vi "GetCurrentPositionDegree.vi"(0 "StepMotor in":refnum<class "StepMotor.lvclass">, 5 "Редукция":dbl, 9 "Разрешение энкодера":dbl, 11 "error in (no error)":errorcluster) -> (4 "StepMotor out":refnum<class "StepMotor.lvclass">, 6 "Значение":dbl, 8 "RawPosition":dbl, 10 "360 и 0":bool, 15 "error out":errorcluster)   [LabVIEW 2010, in "StepMotor.lvclass"]
uses:
  StepMotor.lvclass
panel:
  out "RawPreviousPosition":dbl
  out "МножПриведШкалы360":dbl
  out "КолИмпулОборот":dbl
  out "Текущая позиция":dbl
  out "Инкремент импульсов":dbl
  out "Предыдущая позиция":dbl
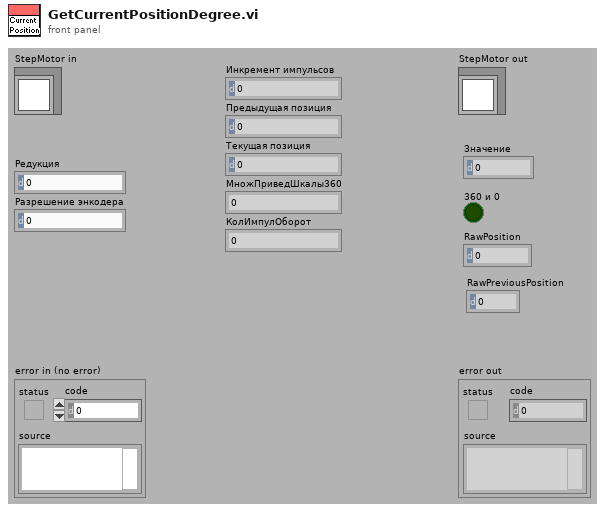
[diagram p1: front panel]
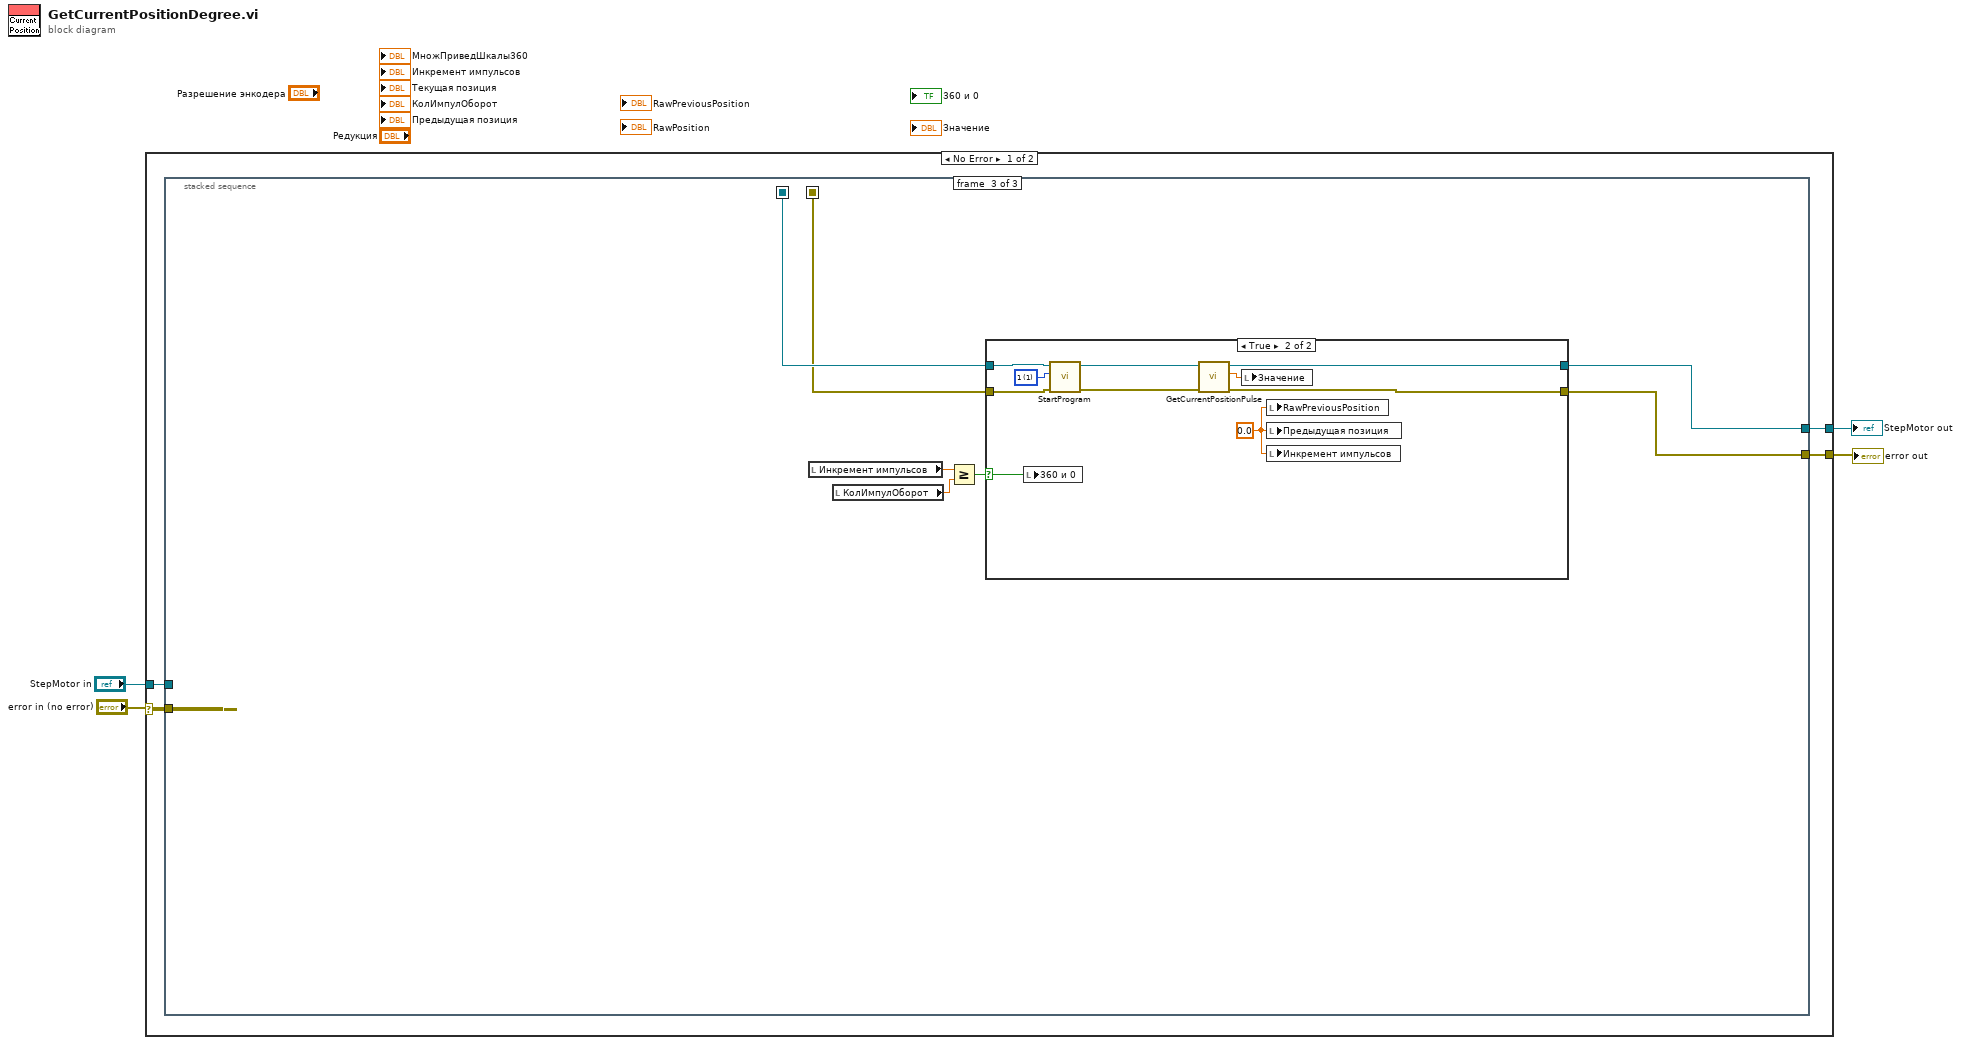
[diagram p0: block diagram]
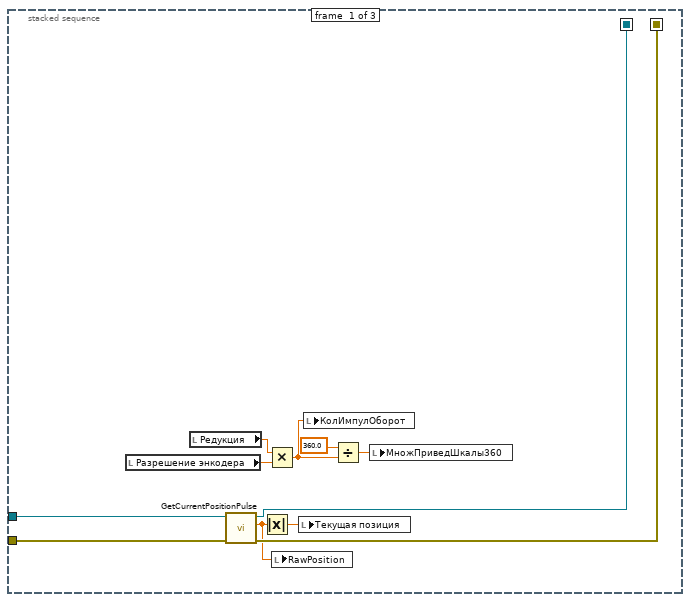
[diagram p2: hidden frame]
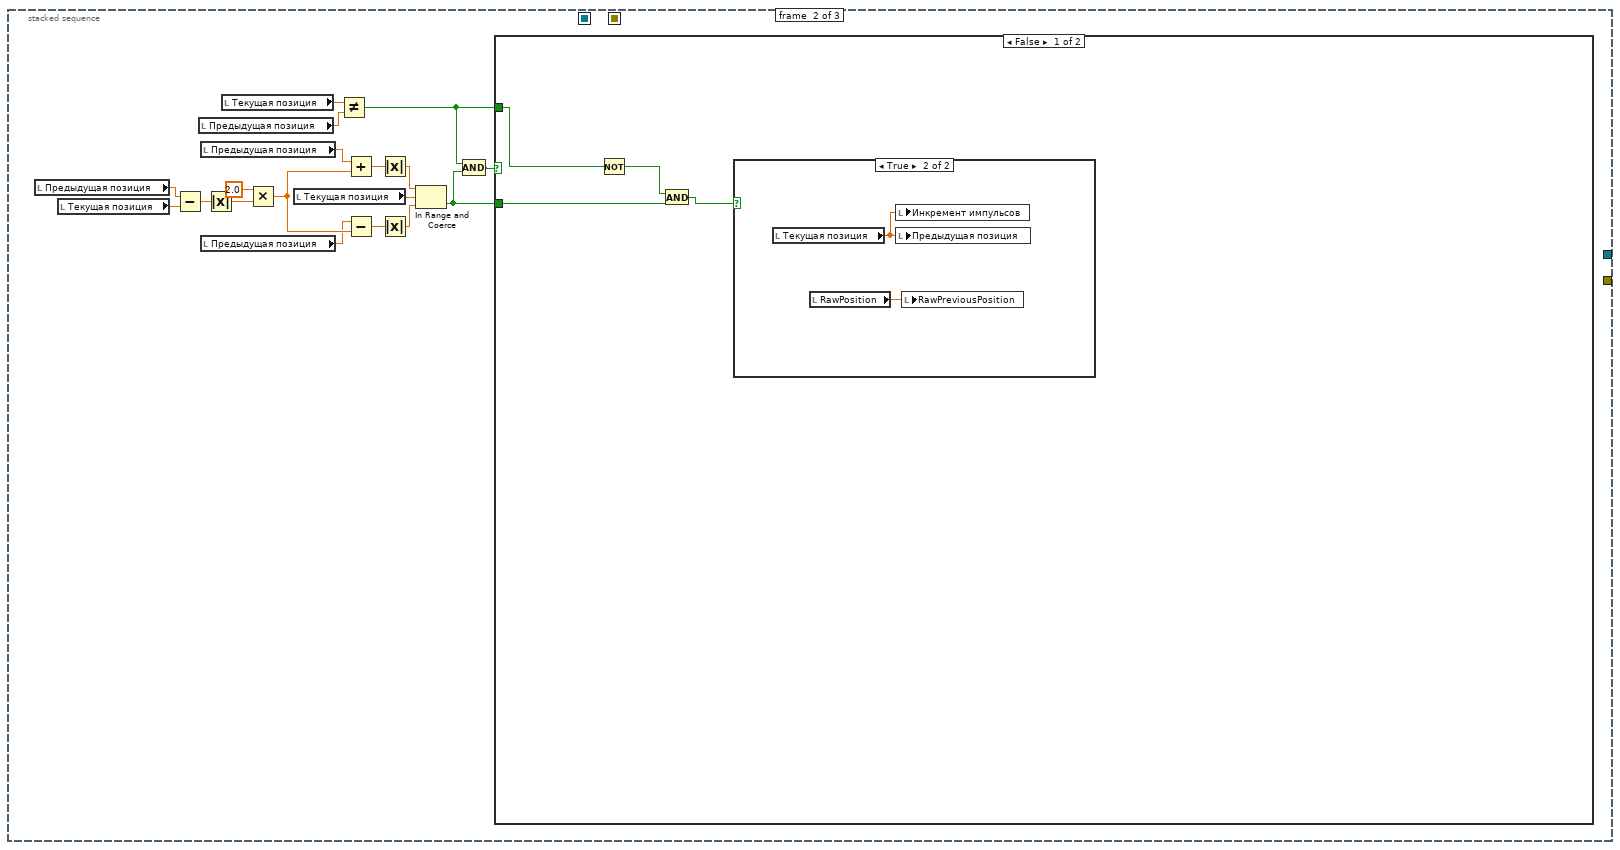
[diagram p3: hidden frame]
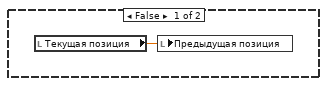
[diagram p4: hidden frame]
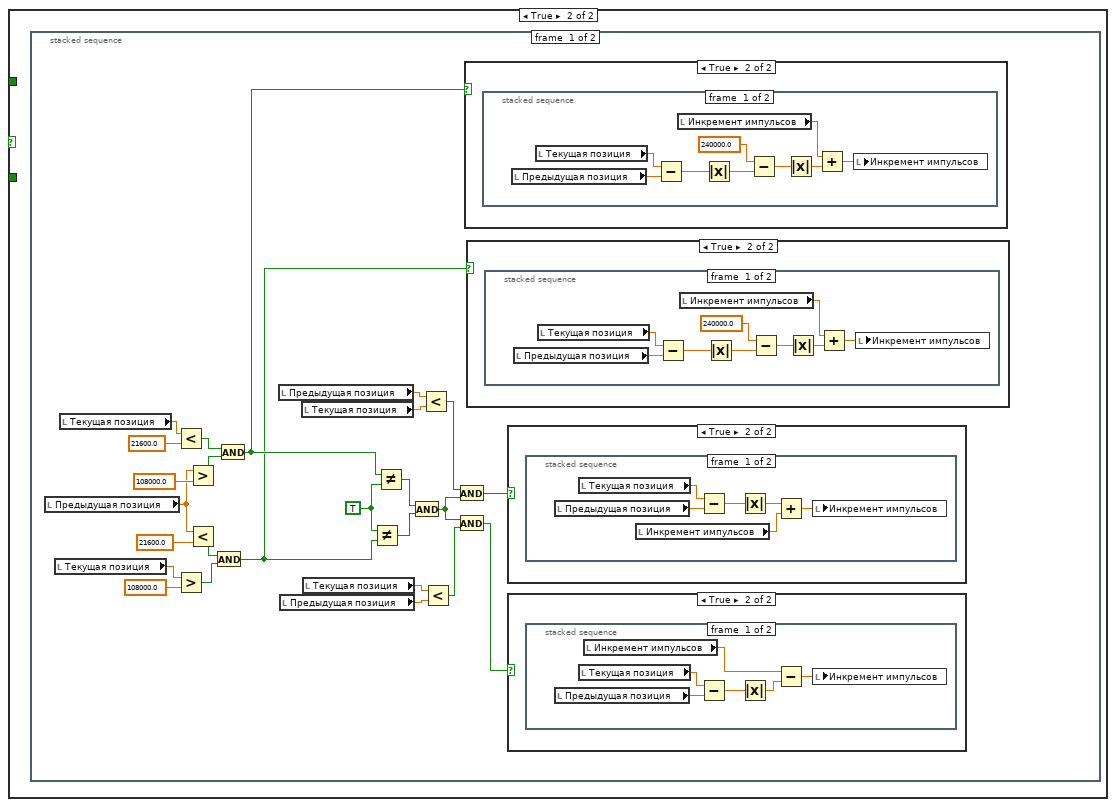
[diagram p5: hidden frame]
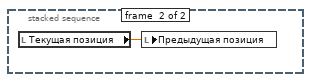
[diagram p7: hidden frame]
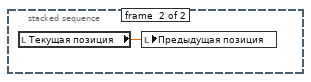
[diagram p9: hidden frame]
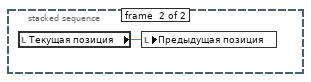
[diagram p11: hidden frame]
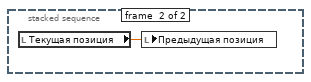
[diagram p13: hidden frame]
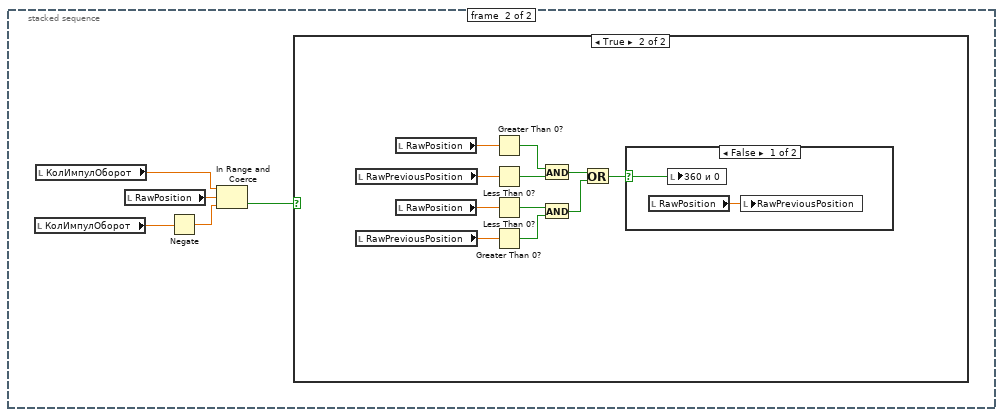
[diagram p14: hidden frame]
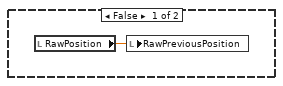
[diagram p15: hidden frame]
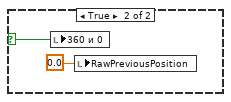
[diagram p16: hidden frame]
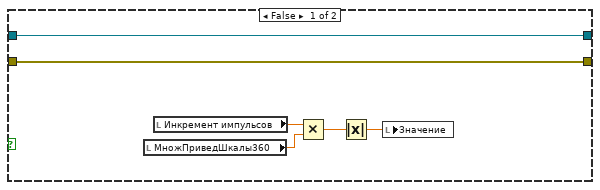
[diagram p17: hidden frame]
diagram:
  n1 = case shown="No Error" "error in (no error)" {
    selector: "error in (no error)" -> [w7 w148]
    tunnel: "StepMotor in" -> [w8 w149]
    tunnel: [w6 w149] -> w1
    tunnel: [w5 w148] -> w2
    frame No Error {
      n2 = stacked-sequence {
        seq-local: [w12 _ _] -> [_ _ w128]
        seq-local: [w11 _ _] -> [_ _ w127]
        tunnel: w8 -> [w14 _ _]
        tunnel: w7 -> [w13 _ _]
        tunnel: [_ _ w126] -> w6
        tunnel: [_ _ w125] -> w5
        frame #0 {
          n3 = local read "Разрешение энкодера"() -> (w18:dbl)
          n4 = local read "Редукция"() -> (w19:dbl)
          n5 = call-dynamic "GetCurrentPositionPulse.vi"("error in (no error)"=w13, "StepMotor in"=w14) -> ("error out"=w11:errorcluster, "Текущая позиция"=w9:dbl, "StepMotor out"=w12:refnum<class "StepMotor.lvclass">)  [unwired: 7 in]
          n6 = Absolute Value(x=w9) -> (abs(x)=w10:dbl)
          n7 = Multiply(x=w19, y=w18) -> (x*y=w16:dbl)
          n8 = local write "RawPosition"(w9) -> ()
          n9 = local write "Текущая позиция"(w10) -> ()
          n10 = local write "КолИмпулОборот"(w16) -> ()
          n11 = Divide(x=360.0, y=w16) -> (x/y=w15:dbl)
          n12 = local write "МножПриведШкалы360"(w15) -> ()
        }
        frame #1 {
          n13 = local read "Предыдущая позиция"() -> (w25:dbl)
          n14 = local read "Текущая позиция"() -> (w28:dbl)
          n15 = Subtract(x=w25, y=w28) -> (x-y=w37:dbl)
          n16 = local read "Предыдущая позиция"() -> (w23:dbl)
          n17 = local read "Предыдущая позиция"() -> (w26:dbl)
          n18 = local read "Предыдущая позиция"() -> (w27:dbl)
          n19 = Absolute Value(x=w37) -> (abs(x)=w35:dbl)
          n20 = local read "Текущая позиция"() -> (w24:dbl)
          n21 = Multiply(x=2.0 ("y"), y=w35) -> (x*y=w34:dbl)
          n22 = local read "Текущая позиция"() -> (w29:dbl)
          n23 = Not Equal?(x=w24, y=w23) -> (x != y?=w20:bool)
          n24 = Add(x=w26, y=w34) -> (x+y=w32:dbl)
          n25 = Subtract(x=w27, y=w34) -> (x-y=w33:dbl)
          n26 = Absolute Value(x=w32) -> (abs(x)=w31:dbl)
          n27 = Absolute Value(x=w33) -> (abs(x)=w30:dbl)
          n28 = In Range and Coerce(upper limit=w31, x=w29, lower limit=w30) -> (In Range?=w21:bool)  [unwired: 1 out]
          n29 = Compound Arithmetic op=AND(w20, w21) -> (w22:bool)
          n30 = case shown="False" w22 {
            tunnel: w21 -> [w39 _]
            tunnel: w20 -> [w41 _]
            frame False {
              n31 = Not(x=w41) -> (.not. x?=w40:bool)
              n32 = And(x=w40, y=w39) -> (x .and. y?=w38:bool)
              n33 = case shown="True" w38 {
                frame False {
                  n34 = local read "Текущая позиция"() -> (w42:dbl)
                  n35 = local write "Предыдущая позиция"(w42) -> ()
                }
                frame True {
                  n36 = local read "Текущая позиция"() -> (w44:dbl)
                  n37 = local read "RawPosition"() -> (w43:dbl)
                  n38 = local write "Инкремент импульсов"(w44) -> ()
                  n39 = local write "Предыдущая позиция"(w44) -> ()
                  n40 = local write "RawPreviousPosition"(w43) -> ()
                }
              }
            }
            frame True {
              n41 = stacked-sequence {
                frame #0 {
                  w60 = TRUE ("x")
                  n42 = local read "Предыдущая позиция"() -> (w67:dbl)
                  n43 = local read "Текущая позиция"() -> (w49:dbl)
                  n44 = local read "Текущая позиция"() -> (w50:dbl)
                  n45 = Less?(x=w50, y=21600.0) -> (x < y?=w63:bool)
                  n46 = Greater?(x=w49, y=108000.0) -> (0:w61:bool)
                  n47 = Greater?(x=w67, y=108000.0) -> (0:w64:bool)
                  n48 = Less?(x=w67, y=21600.0) -> (x < y?=w62:bool)
                  n49 = And(x=w62, y=w61) -> (x .and. y?=w51:bool)
                  n50 = And(x=w63, y=w64) -> (x .and. y?=w52:bool)
                  n51 = local read "Предыдущая позиция"() -> (w56:dbl)
                  n52 = local read "Предыдущая позиция"() -> (w55:dbl)
                  n53 = local read "Текущая позиция"() -> (w48:dbl)
                  n54 = local read "Текущая позиция"() -> (w47:dbl)
                  n55 = Not Equal?(x=w60, y=w51) -> (x != y?=w59:bool)
                  n56 = Not Equal?(x=w52, y=w60) -> (x != y?=w58:bool)
                  n57 = And(x=w58, y=w59) -> (x .and. y?=w57:bool)
                  n58 = Less?(x=w56, y=w48) -> (x < y?=w53:bool)
                  n59 = Less?(x=w47, y=w55) -> (x < y?=w54:bool)
                  n60 = And(x=w53, y=w57) -> (x .and. y?=w45:bool)
                  n61 = And(x=w57, y=w54) -> (x .and. y?=w46:bool)
                  n62 = case shown="True" w52 {
                    frame False {
                    }
                    frame True {
                      n63 = stacked-sequence {
                        frame #0 {
                          n64 = local read "Предыдущая позиция"() -> (w102:dbl)
                          n65 = local read "Текущая позиция"() -> (w94:dbl)
                          n66 = Subtract(x=w94, y=w102) -> (x-y=w101:dbl)
                          n67 = local read "Инкремент импульсов"() -> (w97:dbl)
                          n68 = Absolute Value(x=w101) -> (abs(x)=w100:dbl)
                          n69 = Subtract(x=240000.0, y=w100) -> (x-y=w98:dbl)
                          n70 = Absolute Value(x=w98) -> (abs(x)=w95:dbl)
                          n71 = Add(x=w97, y=w95) -> (x+y=w96:dbl)
                          n72 = local write "Инкремент импульсов"(w96) -> ()
                        }
                        frame #1 {
                          n73 = local read "Текущая позиция"() -> (w103:dbl)
                          n74 = local write "Предыдущая позиция"(w103) -> ()
                        }
                      }
                    }
                  }
                  n75 = case shown="True" w51 {
                    frame False {
                    }
                    frame True {
                      n76 = stacked-sequence {
                        frame #0 {
                          n77 = local read "Предыдущая позиция"() -> (w86:dbl)
                          n78 = local read "Текущая позиция"() -> (w84:dbl)
                          n79 = Subtract(x=w84, y=w86) -> (x-y=w87:dbl)
                          n80 = local read "Инкремент импульсов"() -> (w91:dbl)
                          n81 = Absolute Value(x=w87) -> (abs(x)=w88:dbl)
                          n82 = Subtract(x=240000.0, y=w88) -> (x-y=w90:dbl)
                          n83 = Absolute Value(x=w90) -> (abs(x)=w92:dbl)
                          n84 = Add(x=w91, y=w92) -> (x+y=w85:dbl)
                          n85 = local write "Инкремент импульсов"(w85) -> ()
                        }
                        frame #1 {
                          n86 = local read "Текущая позиция"() -> (w93:dbl)
                          n87 = local write "Предыдущая позиция"(w93) -> ()
                        }
                      }
                    }
                  }
                  n88 = case shown="True" w45 {
                    frame False {
                    }
                    frame True {
                      n89 = stacked-sequence {
                        frame #0 {
                          n90 = local read "Предыдущая позиция"() -> (w82:dbl)
                          n91 = local read "Текущая позиция"() -> (w77:dbl)
                          n92 = local read "Инкремент импульсов"() -> (w79:dbl)
                          n93 = Subtract(x=w77, y=w82) -> (x-y=w80:dbl)
                          n94 = Absolute Value(x=w80) -> (abs(x)=w78:dbl)
                          n95 = Add(x=w78, y=w79) -> (x+y=w81:dbl)
                          n96 = local write "Инкремент импульсов"(w81) -> ()
                        }
                        frame #1 {
                          n97 = local read "Текущая позиция"() -> (w83:dbl)
                          n98 = local write "Предыдущая позиция"(w83) -> ()
                        }
                      }
                    }
                  }
                  n99 = case shown="True" w46 {
                    frame False {
                    }
                    frame True {
                      n100 = stacked-sequence {
                        frame #0 {
                          n101 = local read "Предыдущая позиция"() -> (w75:dbl)
                          n102 = local read "Текущая позиция"() -> (w72:dbl)
                          n103 = local read "Инкремент импульсов"() -> (w71:dbl)
                          n104 = Subtract(x=w72, y=w75) -> (x-y=w73:dbl)
                          n105 = Absolute Value(x=w73) -> (abs(x)=w70:dbl)
                          n106 = Subtract(x=w71, y=w70) -> (x-y=w74:dbl)
                          n107 = local write "Инкремент импульсов"(w74) -> ()
                        }
                        frame #1 {
                          n108 = local read "Текущая позиция"() -> (w76:dbl)
                          n109 = local write "Предыдущая позиция"(w76) -> ()
                        }
                      }
                    }
                  }
                }
                frame #1 {
                  n110 = local read "КолИмпулОборот"() -> (w104:dbl)
                  n111 = local read "КолИмпулОборот"() -> (w105:dbl)
                  n112 = local read "RawPosition"() -> (w108:dbl)
                  n113 = Negate(x=w104) -> (-x=w107:dbl)
                  n114 = In Range and Coerce(upper limit=w105, x=w108, lower limit=w107) -> (In Range?=w106:bool)  [unwired: 1 out]
                  n115 = case shown="True" w106 {
                    frame False {
                      n116 = local read "RawPosition"() -> (w109:dbl)
                      n117 = local write "RawPreviousPosition"(w109) -> ()
                    }
                    frame True {
                      n118 = local read "RawPreviousPosition"() -> (w111:dbl)
                      n119 = local read "RawPreviousPosition"() -> (w113:dbl)
                      n120 = local read "RawPosition"() -> (w110:dbl)
                      n121 = local read "RawPosition"() -> (w112:dbl)
                      n122 = Greater Than 0?(x=w110) -> (x > 0?=w116:bool)
                      n123 = Less Than 0?(x=w111) -> (x < 0?=w117:bool)
                      n124 = Less Than 0?(x=w112) -> (x < 0?=w115:bool)
                      n125 = Greater Than 0?(x=w113) -> (x > 0?=w114:bool)
                      n126 = And(x=w116, y=w117) -> (x .and. y?=w118:bool)
                      n127 = And(x=w115, y=w114) -> (x .and. y?=w119:bool)
                      n128 = Or(x=w118, y=w119) -> (x .or. y?=w120:bool)
                      n129 = case shown="False" w120 {
                        selector: w120 -> [w122 w124]
                        frame False {
                          n130 = local read "RawPosition"() -> (w121:dbl)
                          n131 = local write "360 и 0"(w122) -> ()
                          n132 = local write "RawPreviousPosition"(w121) -> ()
                        }
                        frame True {
                          n133 = local write "360 и 0"(w124) -> ()
                          n134 = local write "RawPreviousPosition"(0.0 ("RawPreviousPosition")) -> ()
                        }
                      }
                    }
                  }
                }
              }
            }
          }
        }
        frame #2 {
          n135 = local read "Инкремент импульсов"() -> (w130:dbl)
          n136 = local read "КолИмпулОборот"() -> (w131:dbl)
          n137 = Greater Or Equal?(x=w130, y=w131) -> (x >= y?=w129:bool)
          n138 = case shown="True" w129 {
            selector: w129 -> [_ w146]
            tunnel: [w133 w145] -> w126
            tunnel: [w132 w144] -> w125
            tunnel: w128 -> [w133 w141]
            tunnel: w127 -> [w132 w140]
            frame False {
              n139 = local read "МножПриведШкалы360"() -> (w134:dbl)
              n140 = local read "Инкремент импульсов"() -> (w135:dbl)
              n141 = Multiply(x=w135, y=w134) -> (x*y=w137:dbl)
              n142 = Absolute Value(x=w137) -> (abs(x)=w136:dbl)
              n143 = local write "Значение"(w136) -> ()
            }
            frame True {
              w142 = 0.0 ("Инкремент импульсов")
              w147 = u16 1 items=["0", "1", "2", "3", "4", "5", "6", "7"] ("Номер банка программ")
              n144 = local write "360 и 0"(w146) -> ()
              n145 = call-dynamic "StartProgram.vi"("error in (no error)"=w140, "Номер банка программ"=w147, "StepMotor in"=w141) -> ("error out"=w138:errorcluster, "StepMotor out"=w139:refnum<class "StepMotor.lvclass">)  [unwired: 7 in]
              n146 = call-dynamic "GetCurrentPositionPulse.vi"("error in (no error)"=w138, "StepMotor in"=w139) -> ("error out"=w144:errorcluster, "Текущая позиция"=w143:dbl, "StepMotor out"=w145:refnum<class "StepMotor.lvclass">)  [unwired: 7 in]
              n147 = local write "Значение"(w143) -> ()
              n148 = local write "RawPreviousPosition"(w142) -> ()
              n149 = local write "Предыдущая позиция"(w142) -> ()
              n150 = local write "Инкремент импульсов"(w142) -> ()
            }
          }
        }
      }
    }
    frame Error {
    }
  }
  "error out" <- w2
  "StepMotor out" <- w1
